vi "Uart Close.vi"(8 "error in (no error)":errorcluster, 10 "Channel":u8, 11 "LMH_LINX in":refnum<class "LINX API.lvclass">) -> (0 "error out":errorcluster, 3 "LMH_LINX out":refnum<class "LINX API.lvclass">)   [LabVIEW 2020, in "LINX API.lvclass"]
uses:
  LINX API.lvclass
  LINX API.lvclass/LINX API.ctl
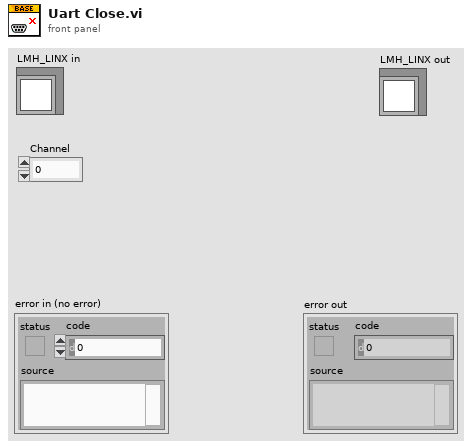
[diagram p1: front panel]
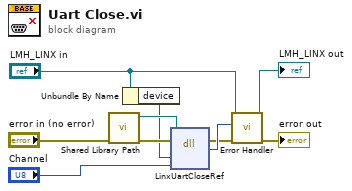
[diagram p0: block diagram]
diagram:
  n1 = call "Shared Library Path.vi"("error in (no error)"="error in (no error)") -> ("error out"=w9:errorcluster, "Path"=w10:path)  [unwired: 9 out]
  n2 = Unbundle By Name("LMH_LINX in") -> ("device"=w2:u64)
  n3 = dll-call lib="Z:/Development/LabVIEW Hobbyist Toolkit/LabVIEW/vi.lib/MakerHub/LINX/Resources/libLinxDevice.dll" fn="LinxUartCloseRef"(path in=w10, error in=w9, "device"=w2, "channel"="Channel") -> (error out=w5:errorcluster, "LinxStatus"=w7:i32)  [unwired: 2 in, 2 out]
  n4 = call "Error Handler.vi"("error in (no error)"=w5, "LINX error code"=w7, "LINX Device"="LMH_LINX in") -> ("error out"=→"error out":errorcluster, "LINX Device out"=→"LMH_LINX out":refnum<class "LINX API.lvclass">)  [unwired: 7 out]
